vi "Send cmd to console and wait for one of many keywords.vi"(5 "Wait msecs after cmd ends (500ms)":u32=500, 6 "VISA resource name":refnum<visa-resource-name>, 7 "Timeout (1000 mSecs)":u32=1000, 8 "error in (no error)":errorcluster, 9 "Wait for keywords":string[](array[string]), 10 "cmd":string, 11 "Wait after send":u32=750) -> (0 "error out":errorcluster, 1 "Response":string, 2 "Keyword found index":i32, 3 "Found key?":bool, 4 "VISA Refnum out":refnum<visa-resource-name>)   [LabVIEW 2024]
uses:
  <vilib>/Utility/error.llb/whitespace.ctl
  <vilib>/Utility/error.llb/Trim Whitespace One-Sided.vi
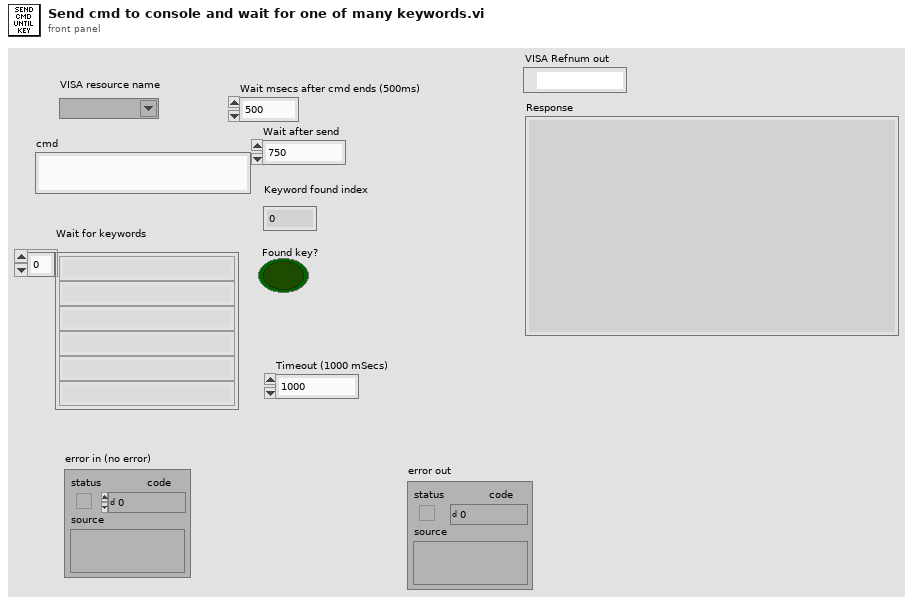
[diagram p1: front panel]
types:
  T1 = typedef "whitespace.ctl" = u16
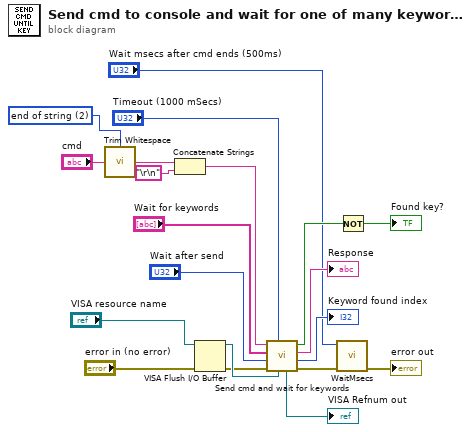
[diagram p0: block diagram]
diagram:
  w9 = T1 2 items=["both", "start of string", "end of string"] ("location (both)")
  n1 = call <vilib>:"Trim Whitespace.vi"("string"="cmd", "location (both)"=w9) -> ("trimmed string"=w7:string)
  n2 = Concatenate Strings(w7, "\r\n") -> (w5:string)
  n3 = VISA Flush I/O Buffer(VISA resource name="VISA resource name", error in (no error)="error in (no error)") -> (VISA resource name out=w3:refnum<visa-resource-name>, error out=w1:errorcluster)  [unwired: 1 in]
  n4 = call "Send cmd and wait for keywords.vi"("VISA resource name"=w3, "Timeout (mSecs)"="Timeout (1000 mSecs)", "error in (no error)"=w1, "Wait after"="Wait after send", "Wait for keywords"="Wait for keywords", "write buffer"=w5) -> ("error out"=w12:errorcluster, "Keyword found index"=→"Keyword found index":i32, "Response"=→"Response":string, "timeout"=w15:bool, "VISA Refnum out"=→"VISA Refnum out":refnum<visa-resource-name>)  [unwired: 1 in]
  n5 = call "WaitMsecs.vi"("error in (no error)"=w12, "Wait Msecs"="Wait msecs after cmd ends (500ms)") -> ("error out"=→"error out":errorcluster)  [unwired: 9 in]
  n6 = Not(x=w15) -> (.not. x?=→"Found key?":bool)
